vi "verify related parameters.vi"(8 "error in (no error)":errorcluster, 11 "Simulated_CCD_Camera in":refnum<class "Simulated_CCD_Camera.lvclass">) -> (0 "error out":errorcluster, 3 "Simulated_CCD_Camera out":refnum<class "Simulated_CCD_Camera.lvclass">)   [LabVIEW 2018, in "Simulated_CCD_Camera.lvclass"]
doc: "Verify the related parameters of the camera\n\nThere are some parameters of the camera operation mode that depend on the value provided for another parameter. This function verifies if these parameters are in agreement."
uses:
  Simulated_CCD_Camera.lvclass
  Simulated_CCD_Camera.lvclass/Simulated_CCD_Camera.ctl
  <vilib>/ErrorRing/Error Ring.xnode
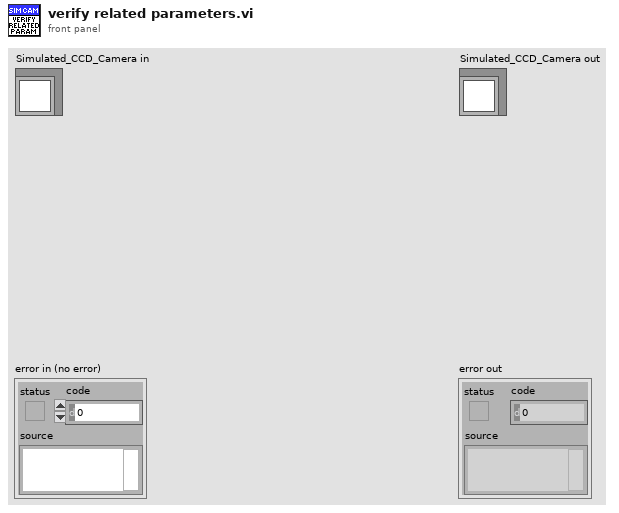
[diagram p1: front panel]
types:
  T1 = cluster{"PREAMP":u16, "READOUT_RATE":u16, "EM_GAIN":u16, "VERTICAL_SHIFT_SPEED":u16, "READ_MODE":u16, "FRAME_TRANSFER":bool, "VERTICAL_CLOCK_VOLTAGE":u16, "ACQUISITION_MODE":u16, "AD_CHANNEL":u16, "EM_MODE":u16, "SHUTTER_TTL":u16, "SHUTTER_OPENING_TIME":u16, "SHUTTER_CLOSING_TIME":u16, "SHUTTER_MODE":u16, "TRIGGER_MODE":u16, "VBIN":u16, "INITIAL_LINE":u16, "INITIAL_COLUMN":u16, "FINAL_LINE":u16, "FINAL_COLUMN":u16, "HBIN":u16}
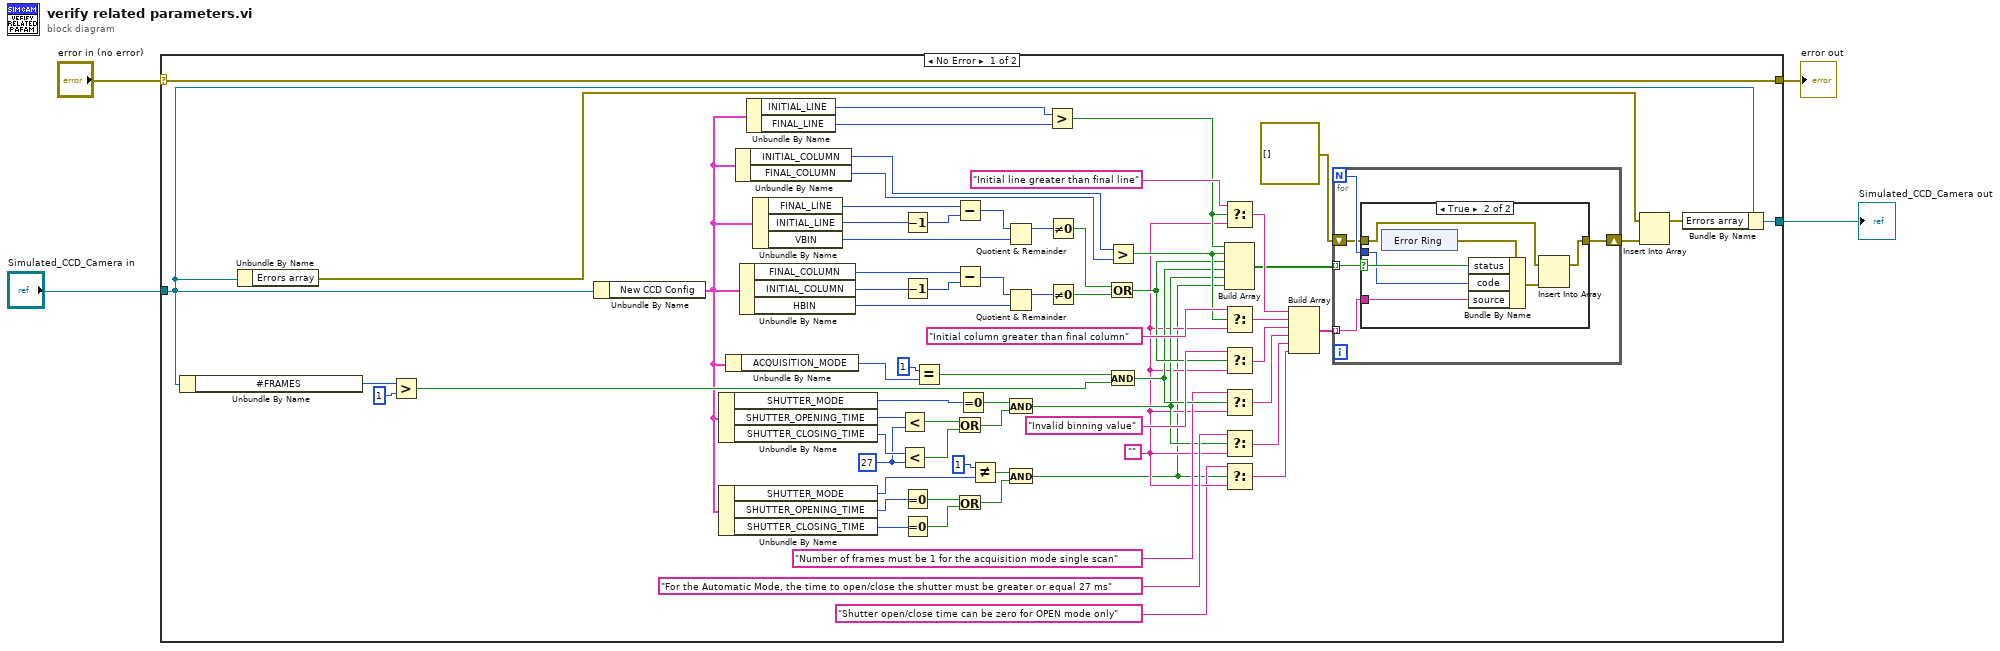
[diagram p0: block diagram]
diagram:
  n1 = case shown="No Error" "error in (no error)" {
    selector: "error in (no error)" -> [w73 w89]
    tunnel: [w73 w89] -> w3
    tunnel: [w11 w88] -> w1
    tunnel: "Simulated_CCD_Camera in" -> [w8 w88]
    frame No Error {
      w30 = 27
      w16 = ""
      n2 = Unbundle By Name(w8) -> ("#FRAMES"=w44:u32)
      n3 = Unbundle By Name(w8) -> ("Errors array"=w7:errorcluster[])
      n4 = Greater?(x=w44, y=1) -> (0:w42:bool)
      n5 = Unbundle By Name(w8) -> ("New CCD Config"=w12:T1)
      n6 = Unbundle By Name(w12) -> ("SHUTTER_MODE"=w34:u16, "SHUTTER_OPENING_TIME"=w32:u16, "SHUTTER_CLOSING_TIME"=w31:u16)
      n7 = Unbundle By Name(w12) -> ("SHUTTER_MODE"=w24:u16, "SHUTTER_OPENING_TIME"=w22:u16, "SHUTTER_CLOSING_TIME"=w21:u16)
      n8 = Unbundle By Name(w12) -> ("ACQUISITION_MODE"=w45:u16)
      n9 = Unbundle By Name(w12) -> ("INITIAL_COLUMN"=w69:u16, "FINAL_COLUMN"=w70:u16)
      n10 = Unbundle By Name(w12) -> ("FINAL_COLUMN"=w52:u16, "INITIAL_COLUMN"=w51:u16, "HBIN"=w50:u16)
      n11 = Unbundle By Name(w12) -> ("INITIAL_LINE"=w72:u16, "FINAL_LINE"=w71:u16)
      n12 = Unbundle By Name(w12) -> ("FINAL_LINE"=w68:u16, "INITIAL_LINE"=w62:u16, "VBIN"=w66:u16)
      n13 = Less?(x=w32, y=w30) -> (x < y?=w29:bool)
      n14 = Less?(x=w31, y=w30) -> (x < y?=w28:bool)
      n15 = Decrement(x=w62) -> (x-1=w61:u16)
      n16 = Decrement(x=w51) -> (x-1=w54:u16)
      n17 = Equal To 0?(x=w22) -> (x = 0?=w20:bool)
      n18 = Equal To 0?(x=w21) -> (x = 0?=w19:bool)
      n19 = Equal?(x=u16 1, y=w45) -> (x = y?=w41:bool)
      n20 = Subtract(x=w68, y=w61) -> (x-y=w67:u16)
      n21 = Subtract(x=w52, y=w54) -> (x-y=w53:u16)
      n22 = Or(x=w29, y=w28) -> (x .or. y?=w27:bool)
      n23 = Or(x=w20, y=w19) -> (x .or. y?=w18:bool)
      n24 = Equal To 0?(x=w34) -> (x = 0?=w33:bool)
      n25 = Not Equal?(x=u16 1, y=w24) -> (x != y?=w17:bool)
      n26 = Quotient & Remainder(x=w67, y=w66) -> (x-y*floor(x/y)=w25:u16)  [unwired: 1 out]
      n27 = Quotient & Remainder(x=w53, y=w50) -> (x-y*floor(x/y)=w46:u16)  [unwired: 1 out]
      n28 = And(x=w33, y=w27) -> (x .and. y?=w26:bool)
      n29 = And(x=w17, y=w18) -> (x .and. y?=w14:bool)
      n30 = Greater?(x=w72, y=w71) -> (0:w57:bool)
      n31 = Not Equal To 0?(x=w25) -> (x != 0?=w48:bool)
      n32 = Not Equal To 0?(x=w46) -> (x != 0?=w47:bool)
      n33 = Or(x=w48, y=w47) -> (x .or. y?=w49:bool)
      n34 = Greater?(x=w69, y=w70) -> (0:w56:bool)
      n35 = And(x=w41, y=w42) -> (x .and. y?=w40:bool)
      n36 = Select(t="Initial line greater than final line", s=w57, f=w16) -> (s? t:f=w60:string)
      n37 = Build Array(w57, w56, w49, w40, w26, w14) -> (w10:bool[])
      n38 = Select(t="Initial column greater than final column", s=w56, f=w16) -> (s? t:f=w59:string)
      n39 = Select(t="Invalid binning value", s=w49, f=w16) -> (s? t:f=w58:string)
      n40 = Select(t="Number of frames must be 1 for the acquisition mode single scan", s=w40, f=w16) -> (s? t:f=w37:string)
      n41 = Select(t="For the Automatic Mode, the time to open/close the shutter must be greater or equal 27 ms", s=w26, f=w16) -> (s? t:f=w36:string)
      n42 = Select(t="Shutter open/close time can be zero for OPEN mode only", s=w14, f=w16) -> (s? t:f=w13:string)
      n43 = Build Array(w60, w59, w58, w37, w36, w13) -> (w55:string[])
      n44 = for {
        N -> [w77]
        tunnel: w55 -> [w76] mode=indexing
        shift-right: [w75] -> w5
        shift-left: errorcluster[] [] -> [w74]
        tunnel: w10 -> [w78] mode=indexing
        n45 = case shown="True" w78 {
          selector: w78 -> [_ w86]
          tunnel: w77 -> [_ w85]
          tunnel: w76 -> [_ w84]
          tunnel: [w79 w83] -> w75
          tunnel: w74 -> [w79 w81]
          frame False {
          }
          frame True {
            n46 = xnode "Error Ring"() -> ("error out"=w82:errorcluster)
            n47 = Bundle By Name(cluster=w82, "status"=w86, "code"=w85, "source"=w84) -> (w80:errorcluster)
            n48 = Insert Into Array(array=w81, new element=w80) -> (w83:errorcluster[])  [unwired: 1 in]
          }
        }
      }
      n49 = Insert Into Array(array=w7, new element=w5) -> (w6:errorcluster[])  [unwired: 1 in]
      n50 = Bundle By Name(cluster=w8, "Errors array"=w6) -> (w11:refnum<class "Simulated_CCD_Camera.lvclass">)
    }
    frame Error {
    }
  }
  "error out" <- w3
  "Simulated_CCD_Camera out" <- w1
